vi "File Path.vi"() -> (2 "File Path":path)   [LabVIEW 2017]
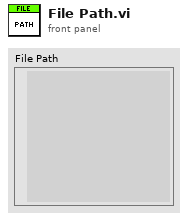
[diagram p1: front panel]
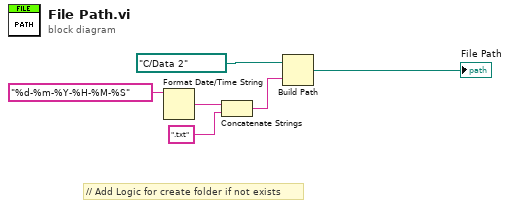
[diagram p0: block diagram]
diagram:
  # "// Add Logic for create folder if not exists"
  n1 = Format Date/Time String(time format string (%c)="%d-%m-%Y-%H-%M-%S") -> (date/time string=w4:string)  [unwired: 2 in]
  n2 = Concatenate Strings(w4, ".txt" ("string")) -> (w5:string)
  n3 = Build Path(base path=path "C:/Data 2", name or relative path=w5) -> (appended path=→"File Path":path)
